vi "sumofphotons.vi"(1 "s":bool, 2 "sum of photons":u32[][][][](array[numeric])) -> (0 "sum of photons out":u32[][][][](array[numeric]))   [LabVIEW 2009]
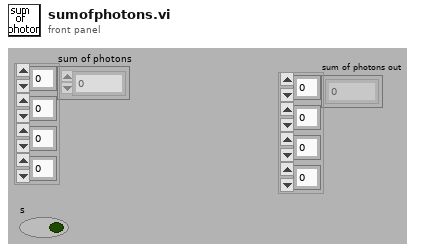
[diagram p1: front panel]
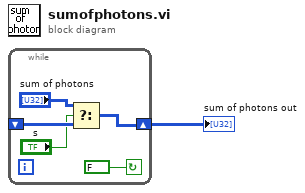
[diagram p0: block diagram]
diagram:
  n1 = while {
    shift-right: [w5] -> w1
    shift-left: _ -> [w4]
    stop <- FALSE continue-if-true
    n2 = Select(t="sum of photons", s="s", f=w4) -> (s? t:f=w5:u32[][][][])
  }
  "sum of photons out" <- w1
